vi "set_status.vi"(8 "error in (no error)":errorcluster, 10 "status":T1, 11 "GenericEmissionSensor.lvclass in":refnum<class "GenericDetector.lvclass">) -> (0 "error out":errorcluster, 3 "GenericEmissionSensor.lvclass out":refnum<class "GenericDetector.lvclass">)   [LabVIEW 2010, in "GenericDetector.lvclass"]
uses:
  GenericDetector.lvclass
  status_enum.ctl
  GenericDetector.lvclass/GenericDetector.ctl
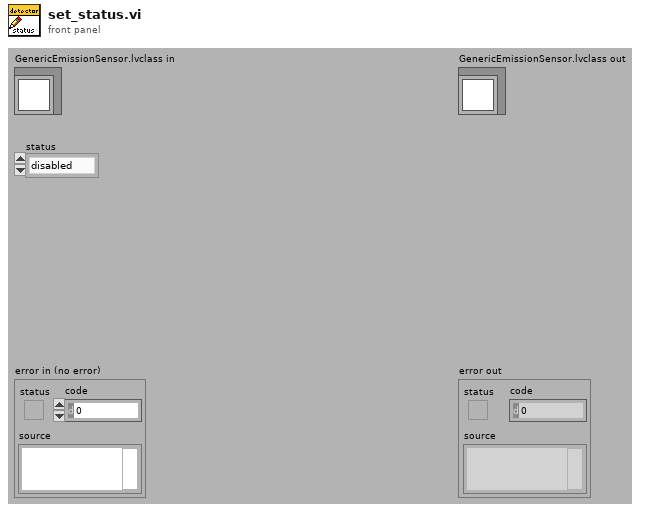
[diagram p1: front panel]
types:
  T1 = typedef "GenericDetector.lvclass/status_enum.ctl" = enum16{"disabled", "enabled"}
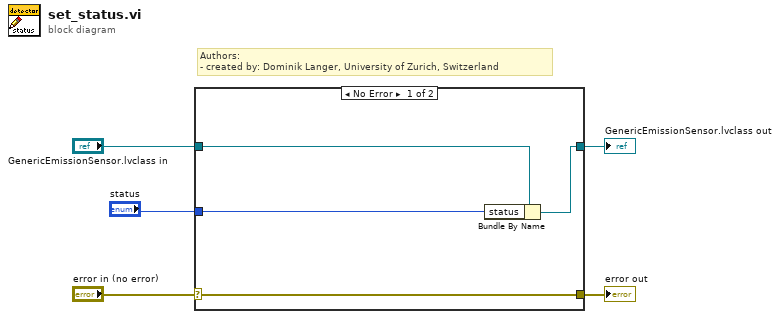
[diagram p0: block diagram]
diagram:
  # "Authors: \n- created by: Dominik Langer, University of Zurich, Switzerland"
  n1 = case shown="No Error" "error in (no error)" {
    selector: "error in (no error)" -> [w9 w10]
    tunnel: [w9 w10] -> w4
    tunnel: [w7 w11] -> w2
    tunnel: "GenericEmissionSensor.lvclass in" -> [w8 w11]
    tunnel: "status" -> [w6 _]
    frame No Error {
      n2 = Bundle By Name(cluster=w8, "status"=w6) -> (w7:refnum<class "GenericDetector.lvclass">)
    }
    frame Error {
    }
  }
  "error out" <- w4
  "GenericEmissionSensor.lvclass out" <- w2
